vi "Example.vi"() -> ()   [LabVIEW 2024]
uses:
  ad903569-9630-40f4-8298-e7330da7f9c3.vi
  99c289bf-7671-4778-adb1-e4095d67b716.vi
  e98ebbe5-6459-453a-9555-421d5fb80c54.vi
  946aa056-9e95-46a1-91c5-935993e4606f.vi
  11e291b6-2fd7-417e-98b3-3ea440b9c247.vi
  TypedCircularBuffer/TypedCircularBuffer.lvclass
  TypedCircularBuffer/Type.ctl
panel:
  out "Full?":bool
  out "Copied Buffer 3":T1[](array[typedef])
  out "Copied Buffer 2":T1[](array[typedef])
  out "Copied Buffer":T1[](array[typedef])
  out "Flushed Buffer 3":T1[](array[typedef])
  out "element":T1
  out "Flushed Buffer":i32[](array[numeric])
  out "Element":i32
  out "CircularBuffer out":T2
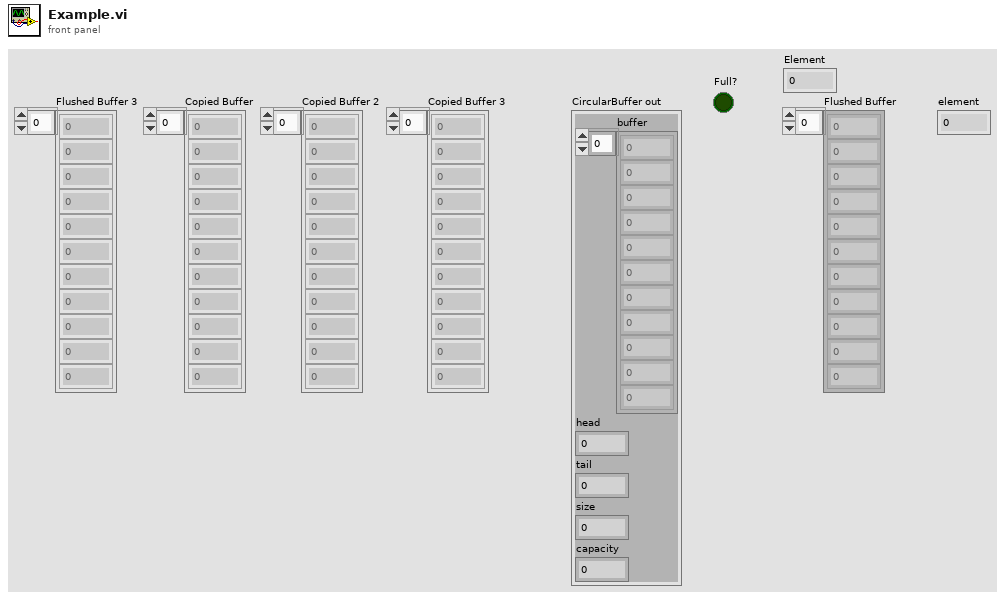
[diagram p1: front panel]
types:
  T1 = typedef "TypedCircularBuffer.lvclass/Type.ctl" = i32
  T2 = cluster{"buffer":i32[], "head":i32, "tail":i32, "size":i32, "capacity":i32}
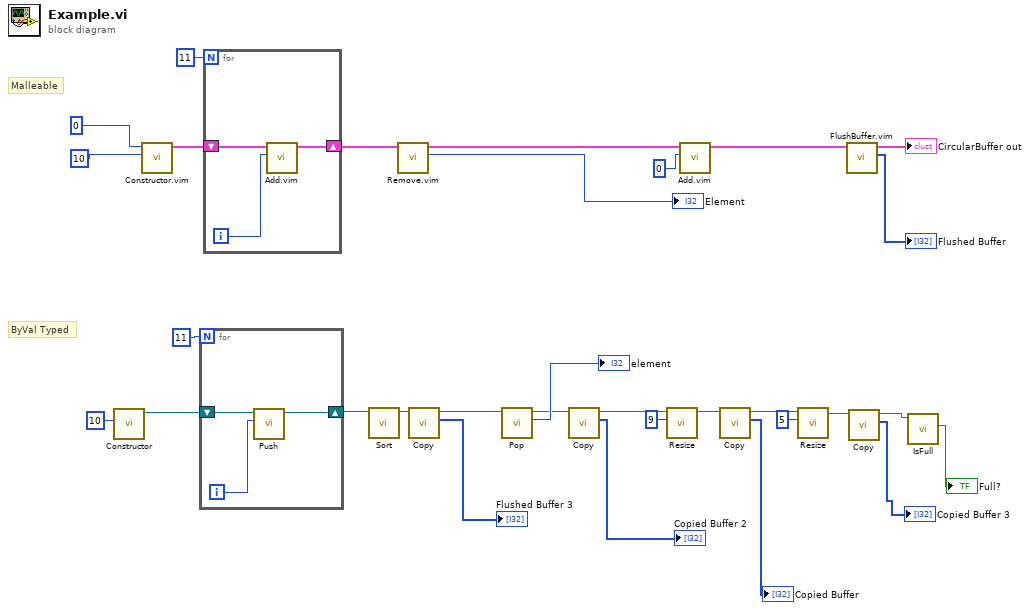
[diagram p0: block diagram]
diagram:
  # "ByVal Typed"
  # "Malleable"
  n1 = call "Constructor.vi"("Capacity"=u32 10) -> ("TypedCircularBuffer out"=w19:refnum<class "TypedCircularBuffer.lvclass">)  [unwired: 10 in]
  n2 = call "Constructor.vim"("Capacity"=10, "Placeholder Type"=0) -> ("CircularBuffer out"=w29:T2)  [unwired: 9 in]
  n3 = for {
    N: 11 -> [_]
    shift-right: [w32] -> w2
    shift-left: w19 -> [w34]
    i -> [w33]
    n4 = call "Push.vi"("Element"=w33, "TypedCircularBuffer in"=w34) -> ("TypedCircularBuffer out"=w32:refnum<class "TypedCircularBuffer.lvclass">)  [unwired: 7 in, 2 out]
  }
  n5 = for {
    N: 11 -> [_]
    shift-right: [w35] -> w27
    shift-left: w29 -> [w37]
    i -> [w36]
    n6 = call "Add.vim"("New Element"=w36, "CircularBuffer in"=w37) -> ("CircularBuffer out"=w35:T2)  [unwired: 7 in, 2 out]
  }
  n7 = call "Sort.vi"("TypedCircularBuffer in"=w2) -> ("TypedCircularBuffer out"=w1:refnum<class "TypedCircularBuffer.lvclass">)  [unwired: 10 in]
  n8 = call "Remove.vim"("CircularBuffer in"=w27) -> ("Element"=→"Element":i32, "CircularBuffer out"=w25:T2)  [unwired: 8 in, 1 out]
  n9 = call "Copy.vi"("TypedCircularBuffer in"=w1) -> ("Copied Buffer"=→"Flushed Buffer 3":T1[], "TypedCircularBuffer out"=w16:refnum<class "TypedCircularBuffer.lvclass">)  [unwired: 9 in]
  n10 = call "Pop.vi"("TypedCircularBuffer in"=w16) -> ("element"=→"element":T1, "TypedCircularBuffer out"=w11:refnum<class "TypedCircularBuffer.lvclass">)  [unwired: 8 in, 1 out]
  n11 = call "Copy.vi"("TypedCircularBuffer in"=w11) -> ("Copied Buffer"=→"Copied Buffer 2":T1[], "TypedCircularBuffer out"=w10:refnum<class "TypedCircularBuffer.lvclass">)  [unwired: 9 in]
  n12 = call "Resize.vi"("Capacity"=u32 9, "TypedCircularBuffer in"=w10) -> ("TypedCircularBuffer out"=w14:refnum<class "TypedCircularBuffer.lvclass">)  [unwired: 9 in]
  n13 = call "Add.vim"("New Element"=0, "CircularBuffer in"=w25) -> ("CircularBuffer out"=w23:T2)  [unwired: 7 in, 2 out]
  n14 = call "Copy.vi"("TypedCircularBuffer in"=w14) -> ("Copied Buffer"=→"Copied Buffer":T1[], "TypedCircularBuffer out"=w7:refnum<class "TypedCircularBuffer.lvclass">)  [unwired: 9 in]
  n15 = call "Resize.vi"("Capacity"=u32 5, "TypedCircularBuffer in"=w7) -> ("TypedCircularBuffer out"=w6:refnum<class "TypedCircularBuffer.lvclass">)  [unwired: 9 in]
  n16 = call "FlushBuffer.vim"("CircularBuffer in"=w23) -> ("Flushed Buffer"=→"Flushed Buffer":i32[], "CircularBuffer out"=→"CircularBuffer out":T2)  [unwired: 9 in]
  n17 = call "Copy.vi"("TypedCircularBuffer in"=w6) -> ("Copied Buffer"=→"Copied Buffer 3":T1[], "TypedCircularBuffer out"=w4:refnum<class "TypedCircularBuffer.lvclass">)  [unwired: 9 in]
  n18 = call "IsFull.vi"("TypedCircularBuffer in"=w4) -> ("Full?"=→"Full?":bool)  [unwired: 9 in, 1 out]
